vi "RemoteFgenSession_CallCloseMeasurementLinkSessionWithCloseBehavior_RemoteSessionClosed.vi"(8 "error in":errorcluster) -> (0 "error out":errorcluster, 2 "result":string, 3 "pass":bool)   [LabVIEW 2020, in "MeasurementServerTests.lvlib"]
uses:
  MeasurementServerTests.lvlib
  Runtime/MeasurementLink Instrument/IInstrument/Close Session Behavior.ctl
  Runtime/MeasurementLink Instrument/IInstrument/IInstrument.lvclass
  Runtime/MeasurementLink niFGEN/Instrument/Instrument.lvclass
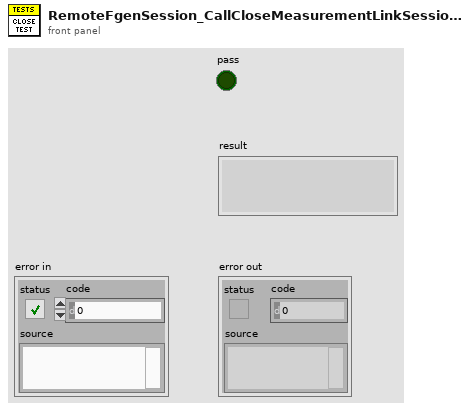
[diagram p1: front panel]
types:
  T1 = typedef "MeasurementLink Instrument.lvlib/IInstrument.lvclass/Remote Connection Options.ctl" = cluster{"session name":string, "address":string, "port":u32}
  T2 = typedef "MeasurementLink Instrument.lvlib/IInstrument.lvclass/Close Session Behavior.ctl" = enum16{"Close Session", "Detach Session"}
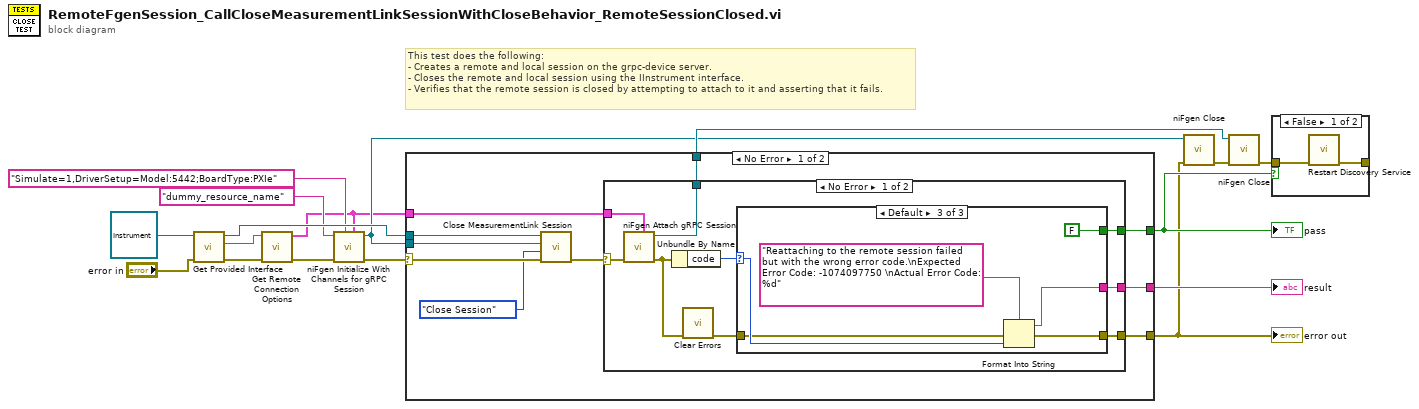
[diagram p0: block diagram]
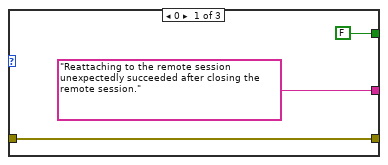
[diagram p3: hidden frame]
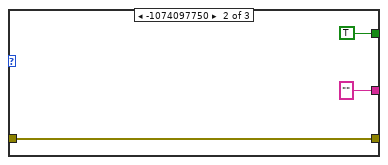
[diagram p4: hidden frame]
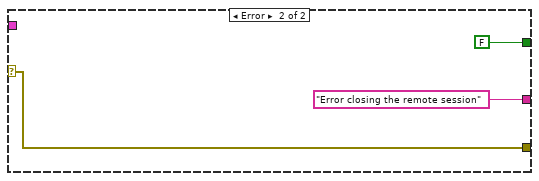
[diagram p5: hidden frame]
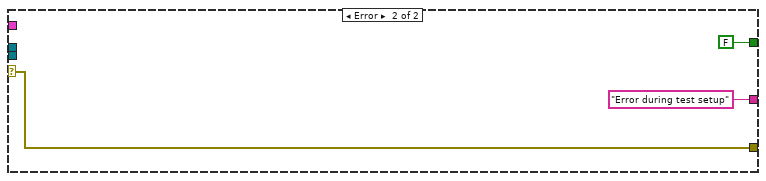
[diagram p6: hidden frame]
diagram:
  # "This test does the following:\n- Creates a remote and local session on the grpc-device server.\n- Closes the remote and local session using the IInstrument interface.\n- Verifies that the remote session is closed by attempting to attach to it and asserting that it fails."
  n1 = call-dynamic "Get Provided Interface.vi"("error in"="error in", "instrument in"=refnum<class "Instrument.lvclass"> refnum ("MeasurementLink niFGEN.lvlib:Instrument.lvclass")) -> ("error out"=w17:errorcluster, "provided interface"=w16:string, "instrument out"=w15:refnum<class "Instrument.lvclass">)  [unwired: 7 in]
  n2 = call "Get Remote Connection Options.vi"("error in"=w17, "provided interface"=w16) -> ("error out"=w6:errorcluster, "remote connection options"=w1:T1)  [unwired: 8 in]
  n3 = call <instrlib>:"niFgen Initialize With Channels for gRPC Session.vi"("gRPC Options"=w1, "Option String"="Simulate=1,DriverSetup=Model:5442;BoardType:PXIe" ("option string"), "error in (no error)"=w6, "Resource Name"="dummy_resource_name" ("resource name")) -> ("error out"=w5:errorcluster, "Instrument Handle Out"=w4:refnum<k15>)  [unwired: 6 in]
  n4 = case shown="No Error" w5 {
    selector: w5 -> [w27 w53]
    tunnel: w15 -> [w26 _]
    tunnel: w4 -> [w25 _]
    tunnel: w1 -> [w24 _]
    tunnel: [w22 w53] -> w8
    tunnel: [w21 FALSE] -> w12
    tunnel: [w20 "Error during test setup" ("f")] -> w13
    tunnel: [w18 _] -> w10
    frame No Error {
      n5 = call-dynamic "Close MeasurementLink Session.vi"("error in"=w27, "close session behavior"=Close_Session_Behavior."Close Session", "session in"=w25, "instrument in"=w26) -> ("error out"=w23:errorcluster)  [unwired: 7 in]
      n6 = case shown="No Error" w23 {
        selector: w23 -> [w36 w49]
        tunnel: w24 -> [w28 _]
        tunnel: [w31 w49] -> w22
        tunnel: [w35 FALSE] -> w21
        tunnel: [w30 "Error closing the remote session" ("f")] -> w20
        tunnel: [w29 _] -> w18
        frame No Error {
          n7 = call <instrlib>:"niFgen Attach gRPC Session.vi"("gRPC Options"=w28, "error in (no error)"=w36) -> ("error out"=w33:errorcluster, "Instrument Handle Out"=w29:refnum<k15>)  [unwired: 8 in]
          n8 = Unbundle By Name(w33) -> ("code"=w34:i32)
          n9 = call <vilib>:"Clear Errors.vi"("error in (no error)"=w33) -> ("error out"=w32:errorcluster)  [unwired: 5 in, 1 out]
          n10 = case shown="Default" w34 {
            selector: w34 -> [_ _ w47]
            tunnel: ["Reattaching to the remote session unexpectedly succeeded after closing the remote session." ("f") "" ("f") w46] -> w30
            tunnel: [FALSE TRUE FALSE] -> w35
            tunnel: w32 -> [w37 w40 w44]
            tunnel: [w37 w40 w43] -> w31
            frame 0 {
            }
            frame -1074097750 {
            }
            frame Default {
              n11 = Format Into String(format string="Reattaching to the remote session failed but with the wrong error code.\nExpected Error Code: -1074097750 \nActual Error Code: %d" ("f"), error in=w44, w47) -> (resulting string=w46:string, error out=w43:errorcluster)  [unwired: 1 in]
            }
          }
        }
        frame Error {
        }
      }
    }
    frame Error {
    }
  }
  "error out" <- w8
  "pass" <- w12
  "result" <- w13
  n12 = call <instrlib>:"niFgen Close.vi"("error in (no error)"=w8, "Instrument Handle"=w4) -> ("error out"=w11:errorcluster)  [unwired: 9 in]
  n13 = call <instrlib>:"niFgen Close.vi"("error in (no error)"=w11, "Instrument Handle"=w10) -> ("error out"=w9:errorcluster)  [unwired: 9 in]
  n14 = case shown="False" w12 {
    tunnel: [w56 _] -> _
    tunnel: w9 -> [w55 _]
    frame False {
      n15 = call "Restart Discovery Service.vi"("error in"=w55) -> ("error out"=w56:errorcluster)  [unwired: 10 in]
    }
    frame True {
    }
  }
